vi "Main.vi"() -> ()   [LabVIEW 2020]
uses:
  <vilib>/platform/TimedLoop/XDataNode/XDataNode.xnode
  <vilib>/Platform/TimedLoop/XDataNode/nitl_modes.ctl
  <vilib>/Platform/TimedLoop/XDataNode/XDNodeRunTimeDep.lvlib
  <vilib>/Platform/TimedLoop/XDataNode/wakeup.ctl
  <vilib>/Platform/TimedLoop/XDataNode/timing_clust.ctl
  <resource>/objmgr/daqmx.rc
  <vilib>/MakerHub/Toolbox/LMH-Toolbox.lvlib
panel:
  in  "Create New File":bool
  out "Output Filename":path
  out "Waveform Chart":waveform(dbl)[](graph)
  in  "Analog Input Mode":enum16{"High Accuracy", "High Speed"}(ring)
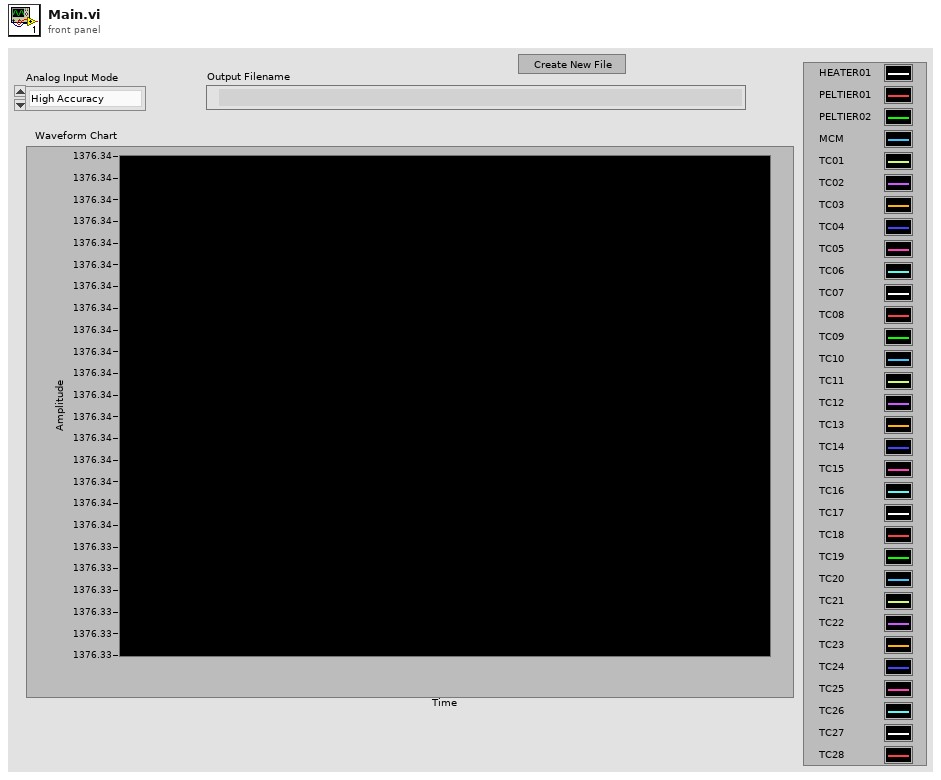
[diagram p1: front panel]
types:
  T1 = typedef "XDNodeRunTimeDep.lvlib/timing_clust.ctl" = cluster{"Expected End [f-1]":u64, "Actual End [f-1]":u64, "Finished Late? [f-1]":bool, "Expected End [i-1]":u64, "Actual End [i-1]":u64, "Finished Late? [i-1]":bool, "Expected Start [i]":u64, "Actual Start [i]":u64, "Expected Start [f]":u64, "Actual Start [f]":u64, "Source Name":string, "Structure Name":string, "Period":i64, "Deadline":i64, "Offset":i64, "Start":i64, "Priority":i32, "Timeout":i32, "Mode":T2, "Wakeup Reason":T3, "Error":errorcluster, "Source Type":string, "Secondary Source Type":string, "Global End Time":u64, "Global Start Time":u64, "Frame Duration":u64, "Iteration Duration":u64, "Assigned CPU":i32, "I/O Scan Engine Mode":u32}
  T2 = typedef "XDNodeRunTimeDep.lvlib/nitl_modes.ctl" = enum32{"No Change", "Process missed periods, maintain original phase", "Discard missed periods, maintain original phase", "Process missed periods, ignore original phase", "Discard missed periods, ignore original phase"}
  T3 = typedef "XDNodeRunTimeDep.lvlib/wakeup.ctl" = enum32{"Normal", "Aborted", "Asynchronous wakeup", "Timing source error", "Timed loop error", "Timeout"}
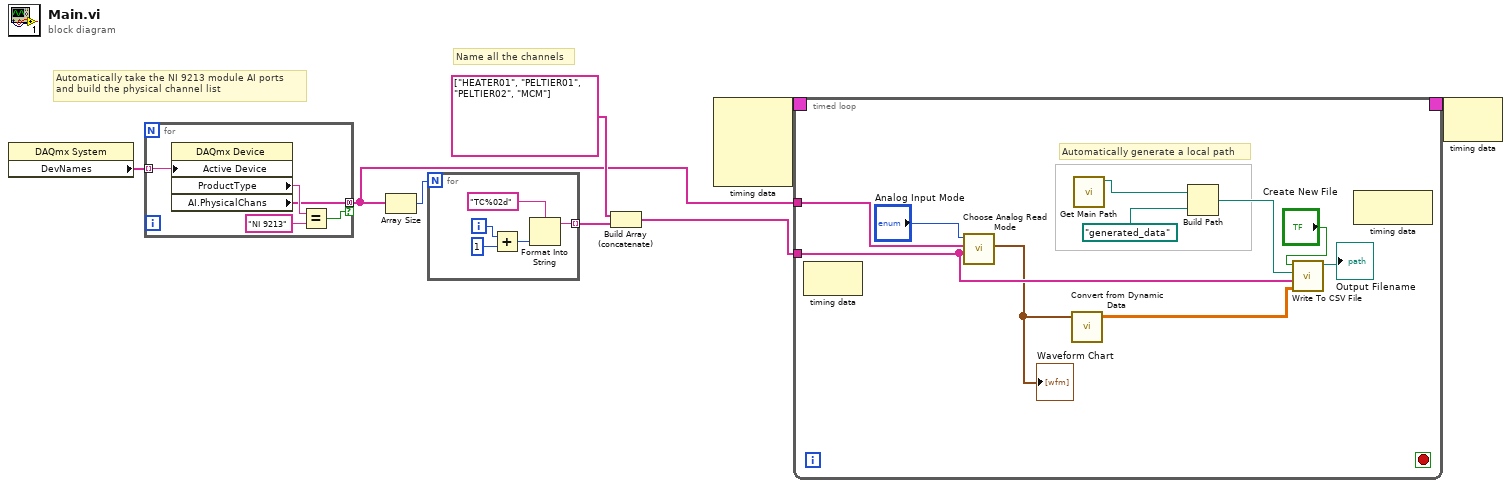
[diagram p0: block diagram]
diagram:
  # "Name all the channels"
  # "Automatically take the NI 9213 module AI ports\nand build the physical channel list"
  n1 = property class="DAQmx System"() -> ("DevNames"=w2:tag[])  [unwired: 2 in, 2 out]
  n2 = for {
    tunnel: w2 -> [w13] mode=indexing
    tunnel: [w10] -> w1 mode=concatenating if=w9
    n3 = property class="DAQmx Device"("Active Device"=w13) -> ("ProductType"=w11:string, "AI.PhysicalChans"=w10:tag[])  [unwired: 2 in, 2 out]
    n4 = Equal?(x=w11, y="NI 9213") -> (x = y?=w9:bool)
  }
  n5 = Array Size(array=w1) -> (size(s)=w8:i32)
  n6 = for {
    N: w8 -> [_]
    tunnel: [w17] -> w7 mode=indexing
    i -> [w16]
    n7 = Add(x=w16, y=1) -> (x+y=w15:i32)
    n8 = Format Into String(format string="TC%02d", w15) -> (resulting string=w17:string)  [unwired: 2 in, 1 out]
  }
  n9 = Build Array (concatenate)(string[] ["HEATER01", "PELTIER01", "PELTIER02", "MCM"], w7) -> (w5:string[])
  n10 = node-c288() -> (w4:T1)  [unwired: 4 in]
  n11 = timed-loop {
    timing: w4 -> [_]
    timing-out: [_] -> w3
    tunnel: w1 -> [w28]
    tunnel: w5 -> [w23]
    stop <- _ stop-if-true
    # "Automatically generate a local path"
    n12 = node-c288() -> ()  [unwired: 1 in, 1 out]
    n13 = call "Choose Analog Read Mode.vi"("Channel Names"=w23, "Physical Channels"=w28, "Analog Input Mode"="Analog Input Mode") -> ("data"=w22:waveform(dbl)[])  [unwired: 8 in]
    "Waveform Chart" <- w22
    n14 = call "Convert from Dynamic Data"("Dynamic Data Type"=w22) -> ("Array"=w21:dbl[][])  [unwired: 3 in]
    n15 = call <vilib>:"Get Main Path.vi"() -> ("Main Dir"=w19:path)  [unwired: 9 in, 2 out]
    n16 = Build Path(base path=w19, name or relative path=path "generated_data") -> (appended path=w24:path)
    n17 = call "Write To CSV File.vi"("Values"=w21, "Names"=w23, "Output Directory"=w24, "Create New File"="Create New File") -> ("Output Filename"=→"Output Filename":path)  [unwired: 7 in]
    n18 = node-c288() -> ()  [unwired: 1 in, 1 out]
  }
  n19 = node-c288(w3) -> ()  [unwired: 1 out]
